vi "Init Master.vi"(7 "Select Layout":refnum<vi>, 8 "error in (no error)":errorcluster, 10 "Trigger Lines":u16[](array[numeric]), 11 "Pulseblaster in":refnum<class "Pulseblaster.lvclass">) -> (0 "error out":errorcluster, 3 "Pulseblaster out":refnum<class "Pulseblaster.lvclass">)   [LabVIEW 2013, in "Pulseblaster.lvclass"]
doc: "Provide simple utility to set up PulseBlaster (all digital colors the same).\nUse ConfigAppearance/Func.vi to safely change ONLY appearance attributes of the device columns.\n\nTriggerLines is an optional input, used by Loading Old setlists, a list of trigger lines in range [0,23]. If this input is provided, any line number appearing in the list will be built as a (disabled) TriggerCol and the user will not be able to modify it in SetList. Otherwise the Trigger Line? control (on the front panel) is used."
uses:
  Pulseblaster.lvclass
  ColumnVIs/Column/Column.lvclass
  ColumnVIs/ModeCol/ModeCol.lvclass
  ColumnVIs/GroupCol/GroupCol.lvclass
  ColumnVIs/DigitalCol/DigitalCol.lvclass
  ColumnVIs/TriggerCol/TriggerCol.lvclass
  TypeDefs/ColumnAppearCluster.ctl
  Globals/DisabledColorGlobal.vi
panel:
  in  "Board Number":i32 max=256 step=1
  in  "SpinAPI Path":path=path "C:/SpinCore/SpinAPI/dll/spinapi.dll"
  in  "Marker Width":u32=30
  in  "Delay Width":u32=30
  in  "Step Width":u32=30
  in  "Comment Width":u32=60
  in  "Mode Width":u32=40
  in  "Gen Text":u32[](array[colorbox])=[0]
  in  "Gen Bkgd":u32[](array[colorbox])=[16771754]
  in  "Group Width":u32=40
  in  "Group Text":u32[](array[colorbox])=[16448250, 0, 0]
  in  "Group Bkgd":u32[](array[colorbox])=[4194432, 10832639, 12880127]
  in  "Digital Width":u32=15
  in  "Dig Text":u32[](array[colorbox])=[16448250, 0, 0]
  in  "Dig Bkgd":u32[](array[colorbox])=[1985280, 6618880, 14090026]
  in  "Trigger Line?":bool[](array[boolean])=[FALSE, FALSE, FALSE, FALSE, FALSE, FALSE, FALSE, FALSE, FALSE, FALSE, FALSE, FALSE, FALSE, FALSE, FALSE, FALSE, FALSE, FALSE, TRUE, TRUE, TRUE, TRUE, TRUE, TRUE]
  # "optional, used by Load Old."
  # "0                          4                          8                         12                        16                        20"
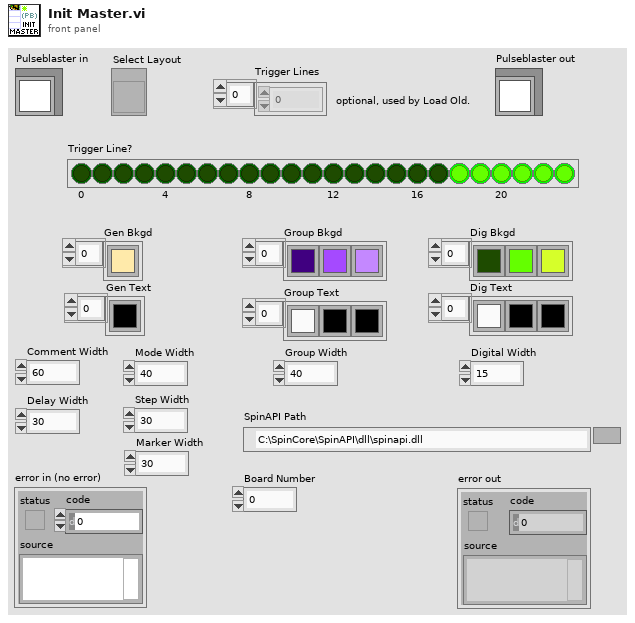
[diagram p1: front panel]
types:
  T1 = typedef "ColumnAppearCluster.ctl" = cluster{"Column Name":string, "Width":u32, "Bkgd":u32[], "Text":u32[]}
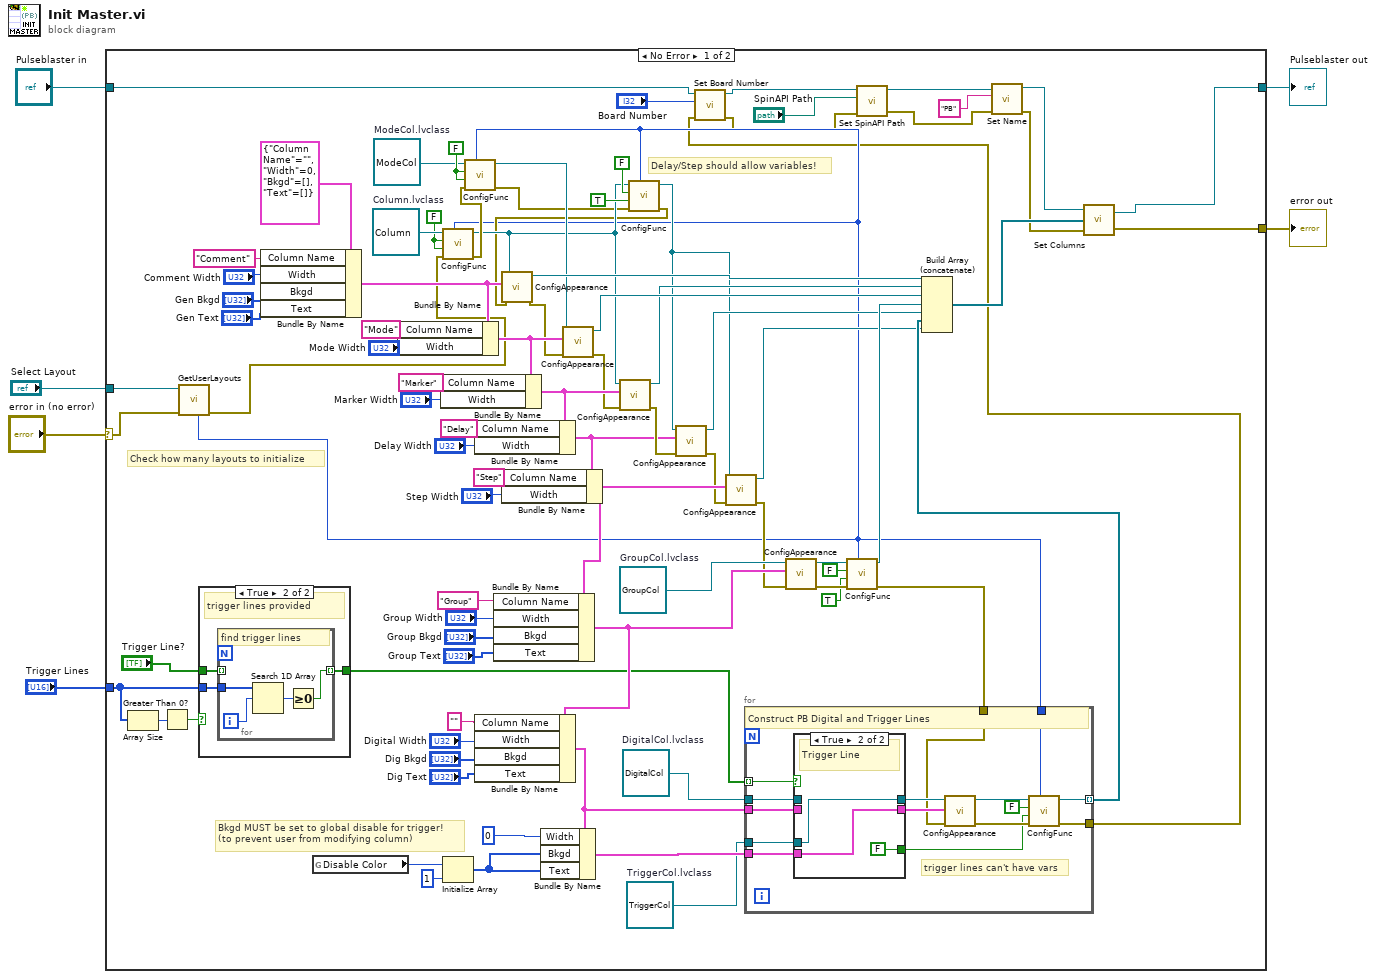
[diagram p0: block diagram]
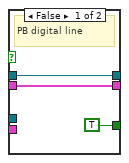
[diagram p3: hidden frame]
diagram:
  n1 = case shown="No Error" "error in (no error)" {
    selector: "error in (no error)" -> [w19 w125]
    tunnel: [w15 w125] -> w5
    tunnel: [w16 w124] -> w3
    tunnel: "Pulseblaster in" -> [w7 w124]
    tunnel: "Trigger Lines" -> [w33 _]
    tunnel: "Select Layout" -> [w20 _]
    frame No Error {
      w41 = FALSE ("Disableable? (True)")
      w42 = FALSE ("Disableable? (True)")
      w59 = refnum<class "DigitalCol.lvclass"> refnum  # DigitalCol.lvclass
      w58 = refnum<class "TriggerCol.lvclass"> refnum  # TriggerCol.lvclass
      w40 = refnum<class "ModeCol.lvclass"> refnum  # ModeCol.lvclass
      w71 = refnum<class "GroupCol.lvclass"> refnum  # GroupCol.lvclass
      w43 = refnum<class "Column.lvclass"> refnum  # Column.lvclass
      # "Delay/Step should allow variables!"
      # "Check how many layouts to initialize"
      # "Bkgd MUST be set to global disable for trigger!\n(to prevent user from modifying column)"
      n2 = Array Size(array=w33) -> (size(s)=w37:i32)
      n3 = Greater Than 0?(x=w37) -> (x > 0?=w34:bool)
      n4 = call "GetUserLayouts.vi"("error in (no error)"=w19, "Layout Ring Refnum"=w20) -> ("error out"=w17:errorcluster, "Num User Layouts"=w18:i32)  [unwired: 5 in, 3 out]
      n5 = case shown="True" w34 {
        tunnel: "Trigger Line?" -> [w95 w98]
        tunnel: [w95 w97] -> w35
        tunnel: w33 -> [_ w96]
        frame False {
          # "Use front panel control"
        }
        frame True {
          # "trigger lines provided"
          n6 = for {
            tunnel: w98 -> [_] mode=indexing
            tunnel: [w99] -> w97 mode=indexing
            tunnel: w96 -> [w102]
            i -> [w101]
            # "find trigger lines"
            n7 = Search 1D Array(1D array=w102, element=w101) -> (index of element=w100:i32)  [unwired: 1 in]
            n8 = Greater Or Equal To 0?(x=w100) -> (x >= 0?=w99:bool)
          }
        }
      }
      n9 = Bundle By Name(cluster=T1 {"Column Name"="", "Width"=0, "Bkgd"=[], "Text"=[]} ("Column Appearance"), "Column Name"="Comment" ("Label (\"\")"), "Width"="Comment Width", "Bkgd"="Gen Bkgd", "Text"="Gen Text") -> (w50:T1)
      n10 = global read "DisabledColorGlobal.vi" "Disable Color"() -> (w65:u32)
      n11 = Bundle By Name(cluster=w50, "Column Name"="Mode" ("Label (\"\")"), "Width"="Mode Width") -> (w77:T1)
      n12 = Bundle By Name(cluster=w77, "Column Name"="Marker" ("Label (\"\")"), "Width"="Marker Width") -> (w78:T1)
      n13 = call "ConfigFunc.vi"("Num Layouts (ignored)"=w18, "error in (no error)"=w17, "isVariable? (True)"=w42, "Disableable? (True)"=w42, "Column in"=w43) -> ("error out"=w38:errorcluster, "Column out"=w24:refnum<class "Column.lvclass">)  [unwired: 5 in]
      n14 = Initialize Array(w65, 1 ("dimension size")) -> (w63:u32[])
      n15 = call "ConfigFunc.vi"("Num Layouts (ignored)"=w18, "error in (no error)"=w38, "isVariable? (True)"=w41, "Disableable? (True)"=w41, "Column in"=w40) -> ("error out"=w22:errorcluster, "Column out"=w39:refnum<class "ModeCol.lvclass">)  [unwired: 5 in]
      n16 = Bundle By Name(cluster=w78, "Column Name"="Delay" ("Label (\"\")"), "Width"="Delay Width") -> (w55:T1)
      n17 = Bundle By Name(cluster=w55, "Column Name"="Step" ("Label (\"\")"), "Width"="Step Width") -> (w54:T1)
      n18 = Bundle By Name(cluster=w54, "Column Name"="Group" ("Label (\"\")"), "Width"="Group Width", "Bkgd"="Group Bkgd", "Text"="Group Text") -> (w66:T1)
      n19 = Bundle By Name(cluster=w66, "Column Name"="" ("Label (\"\")"), "Width"="Digital Width", "Bkgd"="Dig Bkgd", "Text"="Dig Text") -> (w60:T1)
      n20 = Bundle By Name(cluster=w60, "Width"=u32 0 ("Width (60)"), "Bkgd"=w63, "Text"=w63) -> (w61:T1)
      n21 = call "ConfigFunc.vi"("Num Layouts (ignored)"=w18, "error in (no error)"=w22, "isVariable? (True)"=TRUE, "Disableable? (True)"=FALSE, "Column in"=w24) -> ("error out"=w21:errorcluster, "Column out"=w23:refnum<class "Column.lvclass">)  [unwired: 5 in]
      n22 = call "ConfigAppearance.vi"("error in (no error)"=w21, "Column Appearance"=w50, "Column in"=w24) -> ("error out"=w76:errorcluster, "Column out"=w73:refnum<class "Column.lvclass">)  [unwired: 7 in]
      n23 = call "ConfigAppearance.vi"("error in (no error)"=w76, "Column Appearance"=w77, "Column in"=w39) -> ("error out"=w75:errorcluster, "Column out"=w72:refnum<class "ModeCol.lvclass">)  [unwired: 7 in]
      n24 = call "ConfigAppearance.vi"("error in (no error)"=w75, "Column Appearance"=w78, "Column in"=w24) -> ("error out"=w74:errorcluster, "Column out"=w29:refnum<class "Column.lvclass">)  [unwired: 7 in]
      n25 = call "ConfigAppearance.vi"("error in (no error)"=w74, "Column Appearance"=w55, "Column in"=w23) -> ("error out"=w53:errorcluster, "Column out"=w27:refnum<class "Column.lvclass">)  [unwired: 7 in]
      n26 = call "ConfigAppearance.vi"("error in (no error)"=w53, "Column Appearance"=w54, "Column in"=w23) -> ("error out"=w52:errorcluster, "Column out"=w28:refnum<class "Column.lvclass">)  [unwired: 7 in]
      n27 = call "ConfigAppearance.vi"("error in (no error)"=w52, "Column Appearance"=w66, "Column in"=w71) -> ("error out"=w49:errorcluster, "Column out"=w47:refnum<class "GroupCol.lvclass">)  [unwired: 7 in]
      n28 = call "ConfigFunc.vi"("Num Layouts (ignored)"=w18, "error in (no error)"=w49, "isVariable? (True)"=TRUE ("isVariable? (T)"), "Disableable? (True)"=FALSE, "Column in"=w47) -> ("error out"=w48:errorcluster, "Column out"=w46:refnum<class "GroupCol.lvclass">)  [unwired: 5 in]
      n29 = for {
        tunnel: w35 -> [w117] mode=indexing
        tunnel: w61 -> [w116]
        tunnel: w60 -> [w115]
        tunnel: w59 -> [w114]
        tunnel: w58 -> [w113]
        tunnel: [w108] -> w57 mode=indexing
        tunnel: [w106] -> w10
        tunnel: w48 -> [w110]
        tunnel: w18 -> [w103]
        # "trigger lines can't have vars"
        # "Construct PB Digital and Trigger Lines"
        n30 = case shown="True" w117 {
          tunnel: w116 -> [_ w122]
          tunnel: w115 -> [w119 _]
          tunnel: w114 -> [w120 _]
          tunnel: w113 -> [_ w123]
          tunnel: [w120 w123] -> w112
          tunnel: [w119 w122] -> w111
          tunnel: [TRUE FALSE] -> w104
          frame False {
            # "PB digital line"
          }
          frame True {
            # "Trigger Line"
          }
        }
        n31 = call "ConfigAppearance.vi"("error in (no error)"=w110, "Column Appearance"=w111, "Column in"=w112) -> ("error out"=w107:errorcluster, "Column out"=w109:refnum<class "Column.lvclass">)  [unwired: 7 in]
        n32 = call "ConfigFunc.vi"("Num Layouts (ignored)"=w103, "error in (no error)"=w107, "isVariable? (True)"=w104, "Disableable? (True)"=FALSE, "Column in"=w109) -> ("error out"=w106:errorcluster, "Column out"=w108:refnum<class "Column.lvclass">)  [unwired: 5 in]
      }
      n33 = call-dynamic "Set Board Number.vi"("error in (no error)"=w10, "Board Number"="Board Number", "Pulseblaster in"=w7) -> ("error out"=w9:errorcluster, "Pulseblaster out"=w11:refnum<class "Pulseblaster.lvclass">)  [unwired: 7 in]
      n34 = call-dynamic "Set SpinAPI Path.vi"("error in (no error)"=w9, "SpinAPI Path"="SpinAPI Path", "Pulseblaster in"=w11) -> ("error out"=w12:errorcluster, "Pulseblaster out"=w14:refnum<class "Pulseblaster.lvclass">)  [unwired: 7 in]
      n35 = Build Array (concatenate)(w73, w29, w72, w46, w27, w57, w28) -> (w68:refnum<class "Column.lvclass">[])
      n36 = call-dynamic "Set Name.vi"("error in (no error)"=w12, "Name"="PB", "Device in"=w14) -> ("error out"=w67:errorcluster, "Device out"=w94:refnum<class "Pulseblaster.lvclass">)  [unwired: 7 in]
      n37 = call-dynamic "Set Columns.vi"("error in (no error)"=w67, "Columns in"=w68, "Pulseblaster in"=w94) -> ("error out"=w15:errorcluster, "Pulseblaster out"=w16:refnum<class "Pulseblaster.lvclass">)  [unwired: 1 in]
    }
    frame Error {
    }
  }
  "error out" <- w5
  "Pulseblaster out" <- w3
